vi "Define_Place_of_101_Displacement-1.vi"(3 "[IN] Indexes for Jumps":i32[](array[numeric]), 4 "[IN] Subtrack":dbl[](array[numeric]), 5 "[IN] Tracks":dbl[][](array[numeric])) -> (1 "[OUT] Index of \"11\" Dis\nplacement in Subtrack":i32)   [LabVIEW 2013]
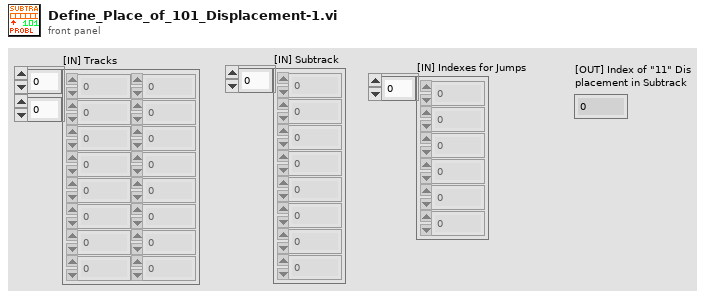
[diagram p1: front panel]
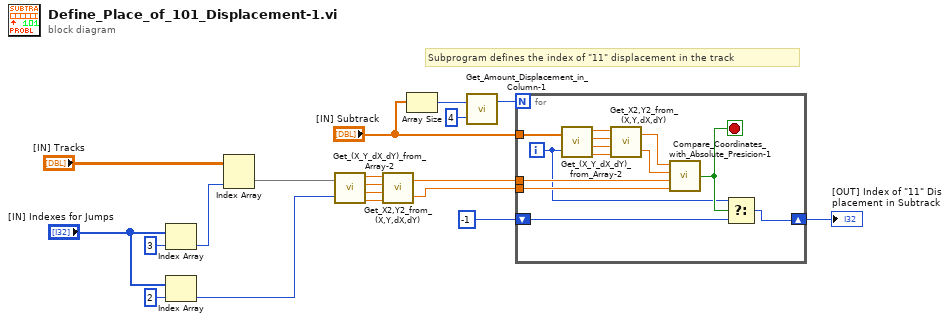
[diagram p0: block diagram]
diagram:
  # "Subprogram defines the index of \"11\" displacement in the track"
  n1 = Index Array(array="[IN] Indexes for Jumps", index=3) -> (element=w17:i32)
  n2 = Index Array(array="[IN] Indexes for Jumps", index=2) -> (element=w13:i32)
  n3 = Index Array(array="[IN] Tracks", index (col)=w17) -> (element=w14:dbl[])  [unwired: 1 in]
  n4 = call "Get_(X_Y_dX_dY)_from_Array-2.vi"("(X,Y,dX,dY)"=w14, "Index of Displacement"=w13) -> ("X"=w6:dbl, "Y"=w5:dbl, "dX"=w4:dbl, "dY"=w3:dbl)
  n5 = call "Get_X2,Y2_from_(X,Y,dX,dY).vi"("dY"=w3, "dX"=w4, "Y1"=w5, "X1"=w6) -> ("Y2 = (Y1+dY)"=w1:dbl, "X2 = (X1+dX)"=w2:dbl)
  n6 = Array Size(array="[IN] Subtrack") -> (size(s)=w12:i32)
  n7 = call "Get_Amount_Displacement_in_Column-1.vi"("multiplier"=4, "# Rows"=w12) -> ("Displ amount"=w10:i32)  [unwired: 1 out]
  n8 = for {
    N: w10 -> [_]
    tunnel: "[IN] Subtrack" -> [w32]
    tunnel: w2 -> [w31]
    tunnel: w1 -> [w30]
    shift-right: [w27] -> w7
    shift-left: -1 -> [w28]
    i -> [w26]
    stop <- w29 stop-if-true
    n9 = call "Get_(X_Y_dX_dY)_from_Array-2.vi"("(X,Y,dX,dY)"=w32, "Index of Displacement"=w26) -> ("X"=w25:dbl, "Y"=w24:dbl, "dX"=w23:dbl, "dY"=w22:dbl)
    n10 = call "Get_X2,Y2_from_(X,Y,dX,dY).vi"("dY"=w22, "dX"=w23, "Y1"=w24, "X1"=w25) -> ("Y2 = (Y1+dY)"=w20:dbl, "X2 = (X1+dX)"=w21:dbl)
    n11 = call "Compare_Coordinates_with_Absolute_Presicion-1.vi"("X 1"=w21, "Y 1"=w20, "X 2"=w31, "Y 2"=w30) -> ("[OUT] Same coordinates?"=w29:bool)  [unwired: 1 in]
    n12 = Select(t=w26, s=w29, f=w28) -> (s? t:f=w27:i32)
  }
  "[OUT] Index of \"11\" Dis\nplacement in Subtrack" <- w7
